vi "StartCapture.vi"(0 "object in":refnum<class "Hamamatsu.lvclass">, 5 "error in (no error)":errorcluster) -> (14 "object out":refnum<class "Hamamatsu.lvclass">, 19 "error out":errorcluster)   [LabVIEW 2021, in "Hamamatsu.lvclass"]
uses:
  Hamamatsu.lvclass
  Hamamatsu.lvclass/Hamamatsu.ctl
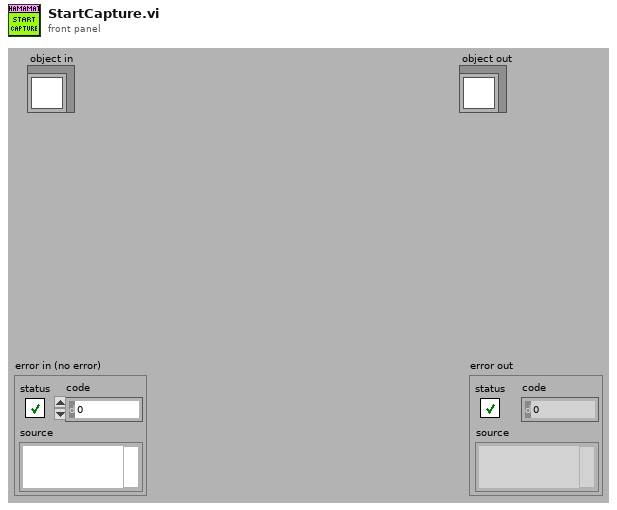
[diagram p1: front panel]
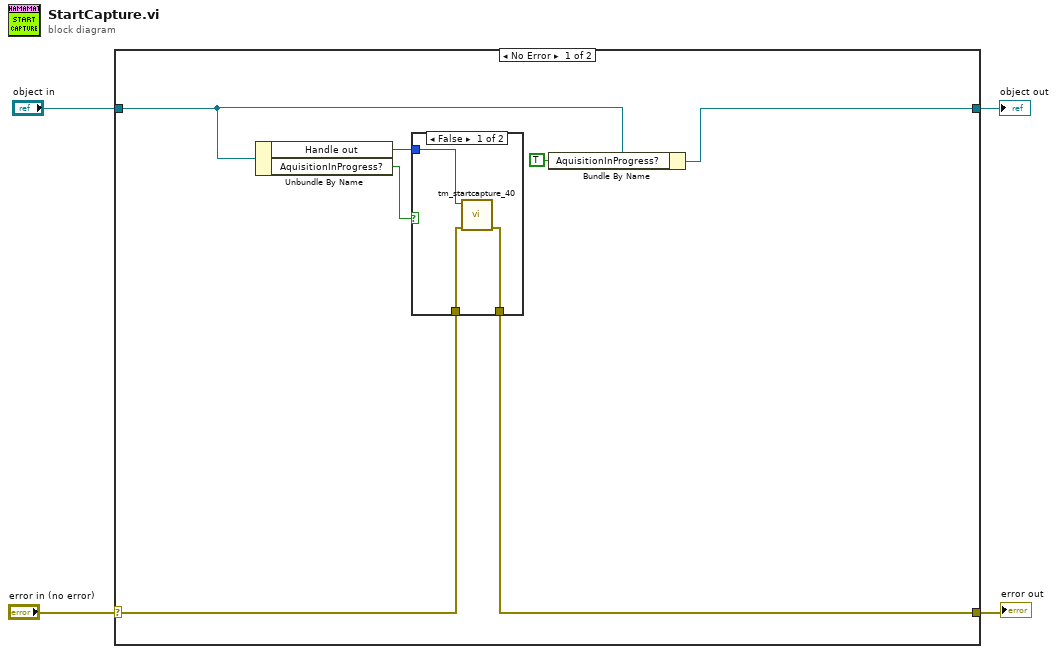
[diagram p0: block diagram]
diagram:
  n1 = case shown="No Error" "error in (no error)" {
    selector: "error in (no error)" -> [w10 w17]
    tunnel: [w9 w17] -> w3
    tunnel: [w8 w16] -> w1
    tunnel: "object in" -> [w7 w16]
    frame No Error {
      n2 = Unbundle By Name(w7) -> ("Handle out"=w11:u32, "AquisitionInProgress?"=w5:bool)
      n3 = case shown="False" w5 {
        tunnel: w11 -> [w14 _]
        tunnel: w10 -> [w13 w15]
        tunnel: [w12 w15] -> w9
        frame False {
          n4 = call <userlib>:"tm_startcapture_40.vi"("error in (no error)"=w13, "Handle in"=w14) -> ("error out"=w12:errorcluster)  [unwired: 8 in, 1 out]
        }
        frame True {
        }
      }
      n5 = Bundle By Name(cluster=w7, "AquisitionInProgress?"=TRUE ("CameraConnected?")) -> (w8:refnum<class "Hamamatsu.lvclass">)
    }
    frame Error {
    }
  }
  "error out" <- w3
  "object out" <- w1
